vi "CSS grouping with jaccard index.vi"() -> ()   [LabVIEW 2014]
uses:
  <vilib>/Utility/file.llb/Read From Spreadsheet File (string).vi
  <vilib>/Utility/file.llb/Write To Spreadsheet File (string).vi
panel:
  in  "save":bool
  in  "file path (to write) 2":path
  in  "cycles":i32=1
  out "Array":string[](array[string])
  in  "cluster centers (original) 7":string[](array[string])=["0 -1 1 -4 0", "0 -1 2 -2 0", "0 -2 3 -3 0", "0 -3 4 -4 0", "0 -1 1 -4 4 -3 0", "0 -1 2 -2 3 -3 0", "0 -4 1 -1 2 -2 0", "0 -4 4 -3 3 -2 0", "0 -1 1 -4 0 -2 3 -3 0", "0 -1 2 -2 0 -4 4 -3 0"]
  out "Assignment (enhanced)":string[](array[string])
  out "Assignment":string[](array[string])
  out "all rows":string[][](array[string])
  in  "cluster centers (original) 5":string[](array[string])=["0 -1 1 -4 0 -4 1 -1 0 -1 1 -4 0 -4 1 -1 0 -1 1 -4 0 -4 1 -1 0 -1 0 -1 1 -4 0 -4 1 -1 0", "0 -1 2 -2 0 -2 2 -1 0 -1 2 -2 0 -2 2 -1 0 -1 2 -2 0 -2 2 -1 0 -1 0 -1 2 -2 0 -2 2 -1 0", "0 -2 3 -3 0 -3 3 -2 0 -2 3 -3 0 -3 3 -2 0 -2 3 -3 0 -3 3 -2 0 -2 0 -2 3 -3 0 -3 3 -2 0", "0 -3 4 -4 0 -4 4 -3 0 -3 4 -4 0 -4 4 -3 0 -3 4 -4 0 -4 4 -3 0 -3 0 -3 4 -4 0 -4 4 -3 0", "0 -1 1 -4 4 -3 0 -3 4 -4 1 -1 0 -1 1 -4 4 -3 0 -3 4 -4 1 -1 0 -1 1 -4 4 -3 0 -3 4 -4 1 -1 0 -1 1 -4 4 -3 0 -3 4 -4 1 -1 0", "0 -1 2 -2 3 -3 0 -3 3 -2 2 -1 0 -1 2 -2 3 -3 0 -3 3 -2 2 -1 0 -1 2 -2 3 -3 0 -3 3 -2 2 -1 0 -1 2 -2 3 -3 0 -3 3 -2 2 -1 0", "0 -4 1 -1 2 -2 0 -2 2 -1 1 -4 0 -4 1 -1 2 -2 0 -2 2 -1 1 -4 0 -4 1 -1 2 -2 0 -2 2 -1 1 -4 0 -4 1 -1 2 -2 0 -2 2 -1 1 -4 0", "0 -4 4 -3 3 -2 0 -2 3 -3 4 -4 0 -4 4 -3 3 -2 0 -2 3 -3 4 -4 0 -4 4 -3 3 -2 0 -2 3 -3 4 -4 0 -4 4 -3 3 -2 0 -2 3 -3 4 -4 0", "0 -1 1 -4 0 -2 3 -3 0 -3 3 -2 0 -4 1 -1 0 -1 1 -4 0 -2 3 -3 0 -3 3 -2 0 -4 1 -1 0 -1 1 -4 0 -2 3 -3 0 -3 3 -2 0 -4 1 -1 0 -1 1 -4 0 -2 3 -3 0 -3 3 -2 0 -4 1 -1 0", "0 -1 2 -2 0 -4 4 -3 0 -3 4 -4 0 -2 2 -1 0 -1 2 -2 0 -4 4 -3 0 -3 4 -4 0 -2 2 -1 0 -1 2 -2 0 -4 4 -3 0 -3 4 -4 0 -2 2 -1 0 -1 2 -2 0 -4 4 -3 0 -3 4 -4 0 -2 2 -1 0"]
  in  "cluster centers (original) 4":string[](array[string])=["0 -1 1 -4 0 -4 1 -1 0 -1 1 -4 0 -4 1 -1 0", "0 -1 2 -2 0 -2 2 -1 0 -1 2 -2 0 -2 2 -1 0", "0 -2 3 -3 0 -3 3 -2 0 -2 3 -3 0 -3 3 -2 0", "0 -3 4 -4 0 -4 4 -3 0 -3 4 -4 0 -4 4 -3 0", "0 -1 1 -4 4 -3 0 -3 4 -4 1 -1 0 -1 1 -4 4 -3 0 -3 4 -4 1 -1 0", "0 -1 2 -2 3 -3 0 -3 3 -2 2 -1 0 -1 2 -2 3 -3 0 -3 3 -2 2 -1 0", "0 -4 1 -1 2 -2 0 -2 2 -1 1 -4 0 -4 1 -1 2 -2 0 -2 2 -1 1 -4 0", "0 -4 4 -3 3 -2 0 -2 3 -3 4 -4 0 -4 4 -3 3 -2 0 -2 3 -3 4 -4 0", "0 -1 1 -4 0 -2 3 -3 0 -3 3 -2 0 -4 1 -1 0 -1 1 -4 0 -2 3 -3 0 -3 3 -2 0 -4 1 -1 0", "0 -1 2 -2 0 -4 4 -3 0 -3 4 -4 0 -2 2 -1 0 -1 2 -2 0 -4 4 -3 0 -3 4 -4 0 -2 2 -1 0"]
  out "size(s)":i32
  in  "cluster centers (original) 3":string[](array[string])=["0 -1 1 -4 0 -4 1 -1 0 -1 1 -4 0 -4 1 -1 0 -1 1 -4 0 -4 1 -1 0", "0 -1 2 -2 0 -2 2 -1 0 -1 2 -2 0 -2 2 -1 0 -1 2 -2 0 -2 2 -1 0", "0 -2 3 -3 0 -3 3 -2 0 -2 3 -3 0 -3 3 -2 0 -2 3 -3 0 -3 3 -2 0", "0 -3 4 -4 0 -4 4 -3 0 -3 4 -4 0 -4 4 -3 0 -3 4 -4 0 -4 4 -3 0", "0 -1 1 -4 4 -3 0 -3 4 -4 1 -1 0 -1 1 -4 4 -3 0 -3 4 -4 1 -1 0 -1 1 -4 4 -3 0 -3 4 -4 1 -1 0", "0 -1 2 -2 3 -3 0 -3 3 -2 2 -1 0 -1 2 -2 3 -3 0 -3 3 -2 2 -1 0 -1 2 -2 3 -3 0 -3 3 -2 2 -1 0", "0 -4 1 -1 2 -2 0 -2 2 -1 1 -4 0 -4 1 -1 2 -2 0 -2 2 -1 1 -4 0 -4 1 -1 2 -2 0 -2 2 -1 1 -4 0", "0 -4 4 -3 3 -2 0 -2 3 -3 4 -4 0 -4 4 -3 3 -2 0 -2 3 -3 4 -4 0 -4 4 -3 3 -2 0 -2 3 -3 4 -4 0", "0 -1 1 -4 0 -2 3 -3 0 -3 3 -2 0 -4 1 -1 0 -1 1 -4 0 -2 3 -3 0 -3 3 -2 0 -4 1 -1 0 -1 1 -4 0 -2 3 -3 0 -3 3 -2 0 -4 1 -1 0", "0 -1 2 -2 0 -4 4 -3 0 -3 4 -4 0 -2 2 -1 0 -1 2 -2 0 -4 4 -3 0 -3 4 -4 0 -2 2 -1 0 -1 2 -2 0 -4 4 -3 0 -3 4 -4 0 -2 2 -1 0"]
  in  "cluster centers (original) 2":string[](array[string])=["0 -1 1 -4 0 -4 1 -1 0", "0 -1 2 -2 0 -2 2 -1 0", "0 -2 3 -3 0 -3 3 -2 0", "0 -3 4 -4 0 -4 4 -3 0", "0 -1 1 -4 4 -3 0 -3 4 -4 1 -1 0", "0 -1 2 -2 3 -3 0 -3 3 -2 2 -1 0", "0 -4 1 -1 2 -2 0 -2 2 -1 1 -4 0", "0 -4 4 -3 3 -2 0 -2 3 -3 4 -4 0", "0 -1 1 -4 0 -2 3 -3 0 -3 3 -2 0 -4 1 -1 0", "0 -1 2 -2 0 -4 4 -3 0 -3 4 -4 0 -2 2 -1 0"]
  out "accuracy":string[][](array[string])
  in  "cluster centers (original) long 5":string[](array[string])=["1 0 -1 1 -1 0 -4 1 -4 0 1 0 -1 1 -1 0 -4 1 -4 0 1 0 -1 1 -1 0 -4 1 -4 0 1 0 -1 1 -1 0 -4 1 -4 0 1 0 -1 1 -1 0 -4 1 -4 0 1", "2 0 -1 2 -1 0 -2 2 -2 0 2 0 -1 2 -1 0 -2 2 -2 0 2 0 -1 2 -1 0 -2 2 -2 0 2 0 -1 2 -1 0 -2 2 -2 0 2 0 -1 2 -1 0 -2 2 -2 0 2", "3 0 -3 3 -3 0 -2 3 -2 0 3 0 -3 3 -3 0 -2 3 -2 0 3 0 -3 3 -3 0 -2 3 -2 0 3 0 -3 3 -3 0 -2 3 -2 0 3 0 -3 3 -3 0 -2 3 -2 0 3", "4 0 -3 4 -3 0 -4 4 -4 0 4 0 -3 4 -3 0 -4 4 -4 0 4 0 -3 4 -3 0 -4 4 -4 0 4 0 -3 4 -3 0 -4 4 -4 0 4 0 -3 4 -3 0 -4 4 -4 0 4", "-1 1 -4 0 -4 4 -3 4 -4 0 -4 1 -1 1 -4 0 -4 4 -3 4 -4 0 -4 1 -1 1 -4 0 -4 4 -3 4 -4 0 -4 1 -1 1 -4 0 -4 4 -3 4 -4 0 -4 1 -1 1 -4 0 -4 4 -3 4 -4 0 -4 1 -1", "-1 2 -2 0 -2 3 -3 3 -2 0 -2 2 -1 2 -2 0 -2 3 -3 3 -2 0 -2 2 -1 2 -2 0 -2 3 -3 3 -2 0 -2 2 -1 2 -2 0 -2 3 -3 3 -2 0 -2 2 -1 2 -2 0 -2 3 -3 3 -2 0 -2 2 -1", "-4 1 -1 0 -1 2 -2 2 -1 0 -1 1 -4 1 -1 0 -1 2 -2 2 -1 0 -1 1 -4 1 -1 0 -1 2 -2 2 -1 0 -1 1 -4 1 -1 0 -1 2 -2 2 -1 0 -1 1 -4 1 -1 0 -1 2 -2 2 -1 0 -1 1 -4", "-4 4 -3 0 -3 3 -2 3 -3 0 -3 4 -4 4 -3 0 -3 3 -2 3 -3 0 -3 4 -4 4 -3 0 -3 3 -2 3 -3 0 -3 4 -4 4 -3 0 -3 3 -2 3 -3 0 -3 4 -4 4 -3 0 -3 3 -2 3 -3 0 -3 4 -4", "0 -4 1 -1 0 -3 3 -2 3 -3 0 -1 1 -4 0 -4 1 -1 0 -3 3 -2 3 -3 0 -1 1 -4 0 -4 1 -1 0 -3 3 -2 3 -3 0 -1 1 -4 0 -4 1 -1 0 -3 3 -2 3 -3 0 -1 1 -4 0 -4 1 -1 0 -3 3 -2 3 -3 0 -1 1 -4 0", "0 -4 4 -3 0 -1 2 -2 2 -1 0 -3 4 -4 0 -4 4 -3 0 -1 2 -2 2 -1 0 -3 4 -4 0 -4 4 -3 0 -1 2 -2 2 -1 0 -3 4 -4 0 -4 4 -3 0 -1 2 -2 2 -1 0 -3 4 -4 0 -4 4 -3 0 -1 2 -2 2 -1 0 -3 4 -4 0"]
  in  "cluster centers (original) long 4":string[](array[string])=["1 0 -1 1 -1 0 -4 1 -4 0 1 0 -1 1 -1 0 -4 1 -4 0 1 0 -1 1 -1 0 -4 1 -4 0 1 0 -1 1 -1 0 -4 1 -4 0 1", "2 0 -1 2 -1 0 -2 2 -2 0 2 0 -1 2 -1 0 -2 2 -2 0 2 0 -1 2 -1 0 -2 2 -2 0 2 0 -1 2 -1 0 -2 2 -2 0 2", "3 0 -3 3 -3 0 -2 3 -2 0 3 0 -3 3 -3 0 -2 3 -2 0 3 0 -3 3 -3 0 -2 3 -2 0 3 0 -3 3 -3 0 -2 3 -2 0 3", "4 0 -3 4 -3 0 -4 4 -4 0 4 0 -3 4 -3 0 -4 4 -4 0 4 0 -3 4 -3 0 -4 4 -4 0 4 0 -3 4 -3 0 -4 4 -4 0 4", "-1 1 -4 0 -4 4 -3 4 -4 0 -4 1 -1 1 -4 0 -4 4 -3 4 -4 0 -4 1 -1 1 -4 0 -4 4 -3 4 -4 0 -4 1 -1 1 -4 0 -4 4 -3 4 -4 0 -4 1 -1", "-1 2 -2 0 -2 3 -3 3 -2 0 -2 2 -1 2 -2 0 -2 3 -3 3 -2 0 -2 2 -1 2 -2 0 -2 3 -3 3 -2 0 -2 2 -1 2 -2 0 -2 3 -3 3 -2 0 -2 2 -1", "-4 1 -1 0 -1 2 -2 2 -1 0 -1 1 -4 1 -1 0 -1 2 -2 2 -1 0 -1 1 -4 1 -1 0 -1 2 -2 2 -1 0 -1 1 -4 1 -1 0 -1 2 -2 2 -1 0 -1 1 -4", "-4 4 -3 0 -3 3 -2 3 -3 0 -3 4 -4 4 -3 0 -3 3 -2 3 -3 0 -3 4 -4 4 -3 0 -3 3 -2 3 -3 0 -3 4 -4 4 -3 0 -3 3 -2 3 -3 0 -3 4 -4", "0 -4 1 -1 0 -3 3 -2 3 -3 0 -1 1 -4 0 -4 1 -1 0 -3 3 -2 3 -3 0 -1 1 -4 0 -4 1 -1 0 -3 3 -2 3 -3 0 -1 1 -4 0 -4 1 -1 0 -3 3 -2 3 -3 0 -1 1 -4 0", "0 -4 4 -3 0 -1 2 -2 2 -1 0 -3 4 -4 0 -4 4 -3 0 -1 2 -2 2 -1 0 -3 4 -4 0 -4 4 -3 0 -1 2 -2 2 -1 0 -3 4 -4 0 -4 4 -3 0 -1 2 -2 2 -1 0 -3 4 -4 0"]
  in  "cluster centers (original) long 3":string[](array[string])=["1 0 -1 1 -1 0 -4 1 -4 0 1 0 -1 1 -1 0 -4 1 -4 0 1 0 -1 1 -1 0 -4 1 -4 0 1", "2 0 -1 2 -1 0 -2 2 -2 0 2 0 -1 2 -1 0 -2 2 -2 0 2 0 -1 2 -1 0 -2 2 -2 0 2", "3 0 -3 3 -3 0 -2 3 -2 0 3 0 -3 3 -3 0 -2 3 -2 0 3 0 -3 3 -3 0 -2 3 -2 0 3", "4 0 -3 4 -3 0 -4 4 -4 0 4 0 -3 4 -3 0 -4 4 -4 0 4 0 -3 4 -3 0 -4 4 -4 0 4", "-1 1 -4 0 -4 4 -3 4 -4 0 -4 1 -1 1 -4 0 -4 4 -3 4 -4 0 -4 1 -1 1 -4 0 -4 4 -3 4 -4 0 -4 1 -1", "-1 2 -2 0 -2 3 -3 3 -2 0 -2 2 -1 2 -2 0 -2 3 -3 3 -2 0 -2 2 -1 2 -2 0 -2 3 -3 3 -2 0 -2 2 -1", "-4 1 -1 0 -1 2 -2 2 -1 0 -1 1 -4 1 -1 0 -1 2 -2 2 -1 0 -1 1 -4 1 -1 0 -1 2 -2 2 -1 0 -1 1 -4", "-4 4 -3 0 -3 3 -2 3 -3 0 -3 4 -4 4 -3 0 -3 3 -2 3 -3 0 -3 4 -4 4 -3 0 -3 3 -2 3 -3 0 -3 4 -4", "0 -4 1 -1 0 -3 3 -2 3 -3 0 -1 1 -4 0 -4 1 -1 0 -3 3 -2 3 -3 0 -1 1 -4 0 -4 1 -1 0 -3 3 -2 3 -3 0 -1 1 -4 0", "0 -4 4 -3 0 -1 2 -2 2 -1 0 -3 4 -4 0 -4 4 -3 0 -1 2 -2 2 -1 0 -3 4 -4 0 -4 4 -3 0 -1 2 -2 2 -1 0 -3 4 -4 0"]
  in  "cluster centers (original) long":string[](array[string])=["1 0 -1 1 -1 0 -4 1 -4 0 1 0 -1 1 -1 0 -4 1 -4 0 1", "2 0 -1 2 -1 0 -2 2 -2 0 2 0 -1 2 -1 0 -2 2 -2 0 2", "3 0 -3 3 -3 0 -2 3 -2 0 3 0 -3 3 -3 0 -2 3 -2 0 3", "4 0 -3 4 -3 0 -4 4 -4 0 4 0 -3 4 -3 0 -4 4 -4 0 4", "-1 1 -4 0 -4 4 -3 4 -4 0 -4 1 -1 1 -4 0 -4 4 -3 4 -4 0 -4 1 -1", "-1 2 -2 0 -2 3 -3 3 -2 0 -2 2 -1 2 -2 0 -2 3 -3 3 -2 0 -2 2 -1", "-4 1 -1 0 -1 2 -2 2 -1 0 -1 1 -4 1 -1 0 -1 2 -2 2 -1 0 -1 1 -4", "-4 4 -3 0 -3 3 -2 3 -3 0 -3 4 -4 4 -3 0 -3 3 -2 3 -3 0 -3 4 -4", "0 -4 1 -1 0 -3 3 -2 3 -3 0 -1 1 -4 0 -4 1 -1 0 -3 3 -2 3 -3 0 -1 1 -4 0", "0 -4 4 -3 0 -1 2 -2 2 -1 0 -3 4 -4 0 -4 4 -3 0 -1 2 -2 2 -1 0 -3 4 -4 0"]
  out "Results":string[][](array[string])
  in  "file path (dialog if empty)":path=path "K:/PhD work/PhD research work 2/Common substring validation/documentation/Data final results/Common substrings (ground truth 2 CHECKED).txt"
  in  "cluster centers (original)":string[](array[string])=["1 0 -1 1 -1 0 -4 1 -4 0 1", "2 0 -1 2 -1 0 -2 2 -2 0 2", "3 0 -3 3 -3 0 -2 3 -2 0 3", "4 0 -3 4 -3 0 -4 4 -4 0 4", "-1 1 -4 0 -4 4 -3 4 -4 0 -4 1 -1", "-1 2 -2 0 -2 3 -3 3 -2 0 -2 2 -1", "-4 1 -1 0 -1 2 -2 2 -1 0 -1 1 -4", "-4 4 -3 0 -3 3 -2 3 -3 0 -3 4 -4", "0 -4 1 -1 0 -3 3 -2 3 -3 0 -1 1 -4 0", "0 -4 4 -3 0 -1 2 -2 2 -1 0 -3 4 -4 0"]
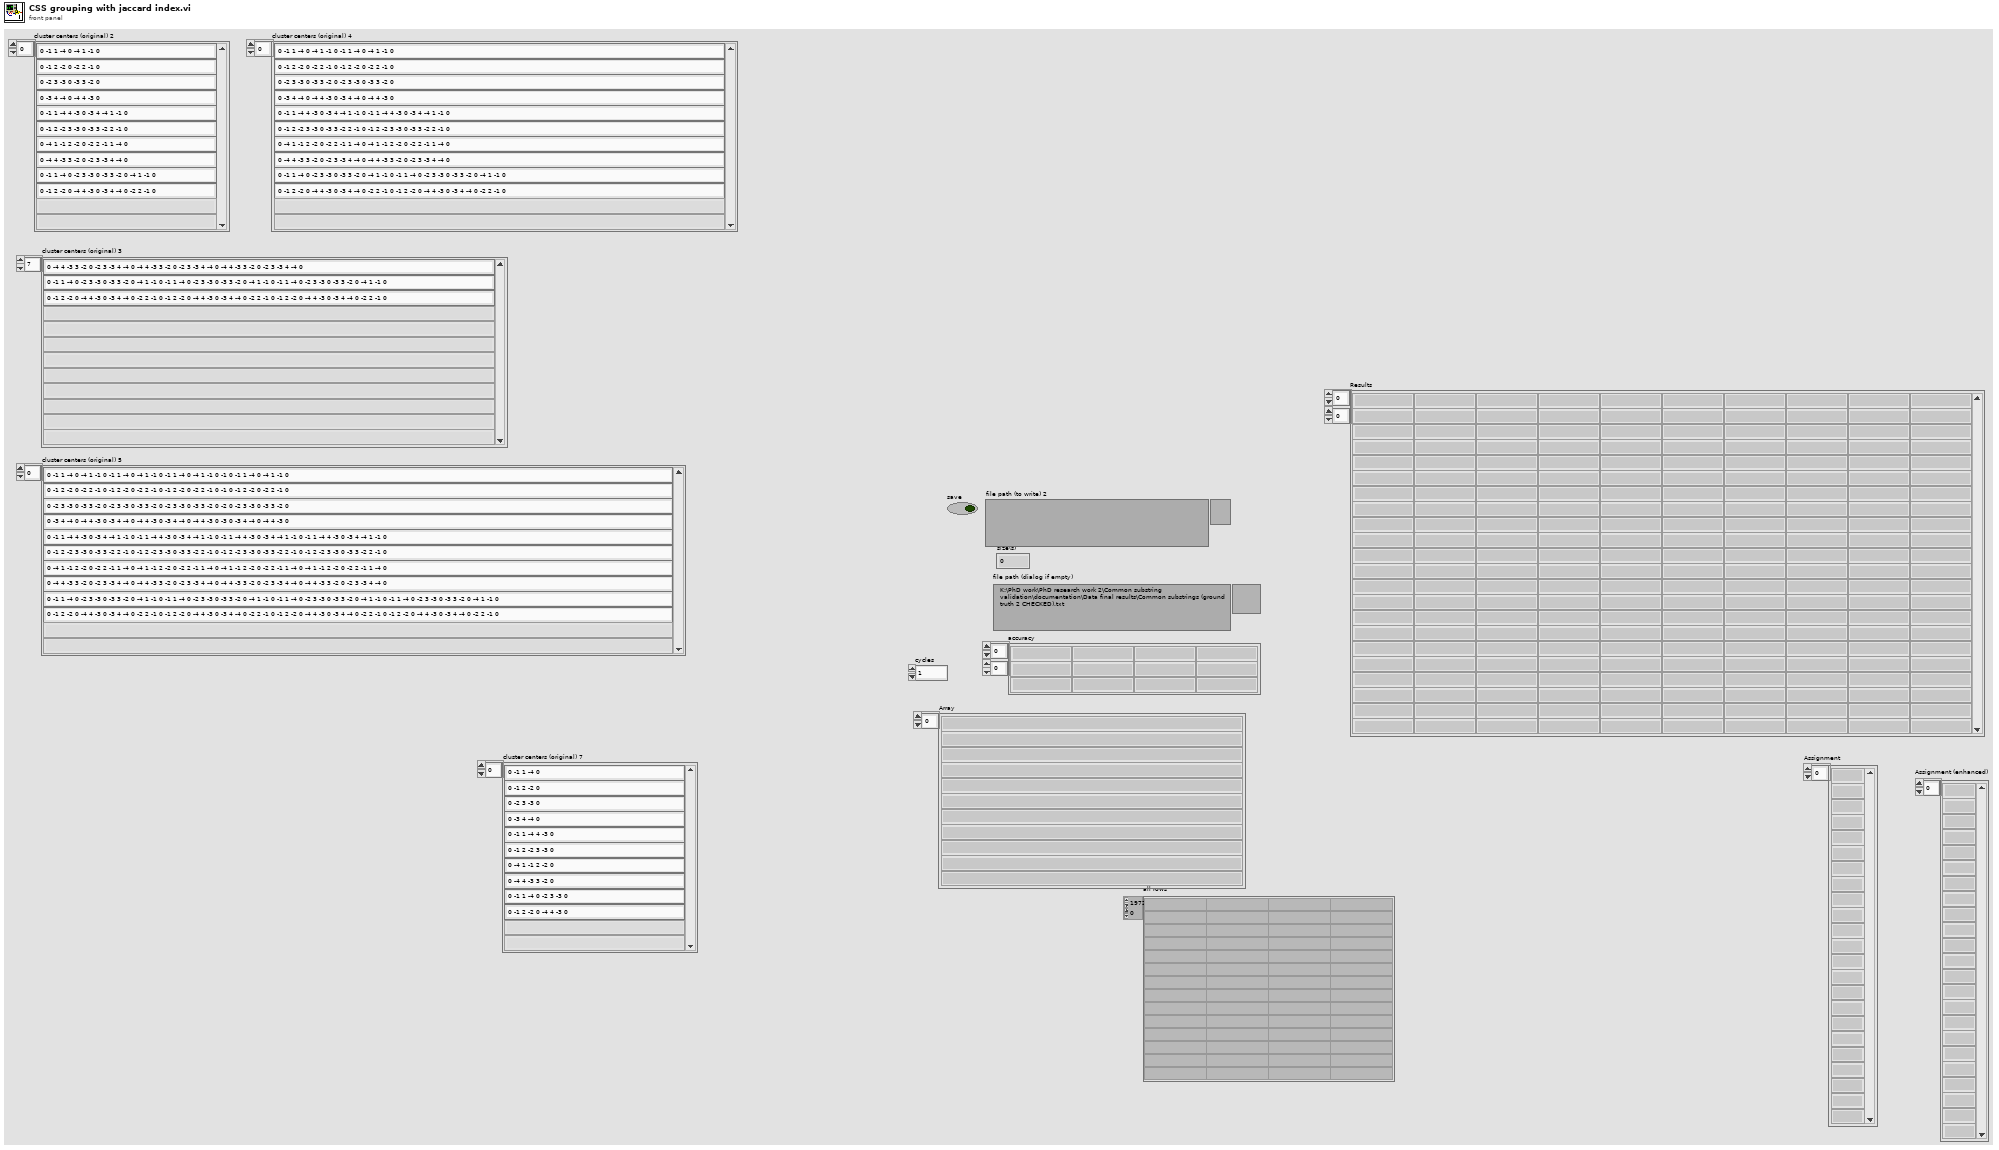
[diagram p1: front panel]
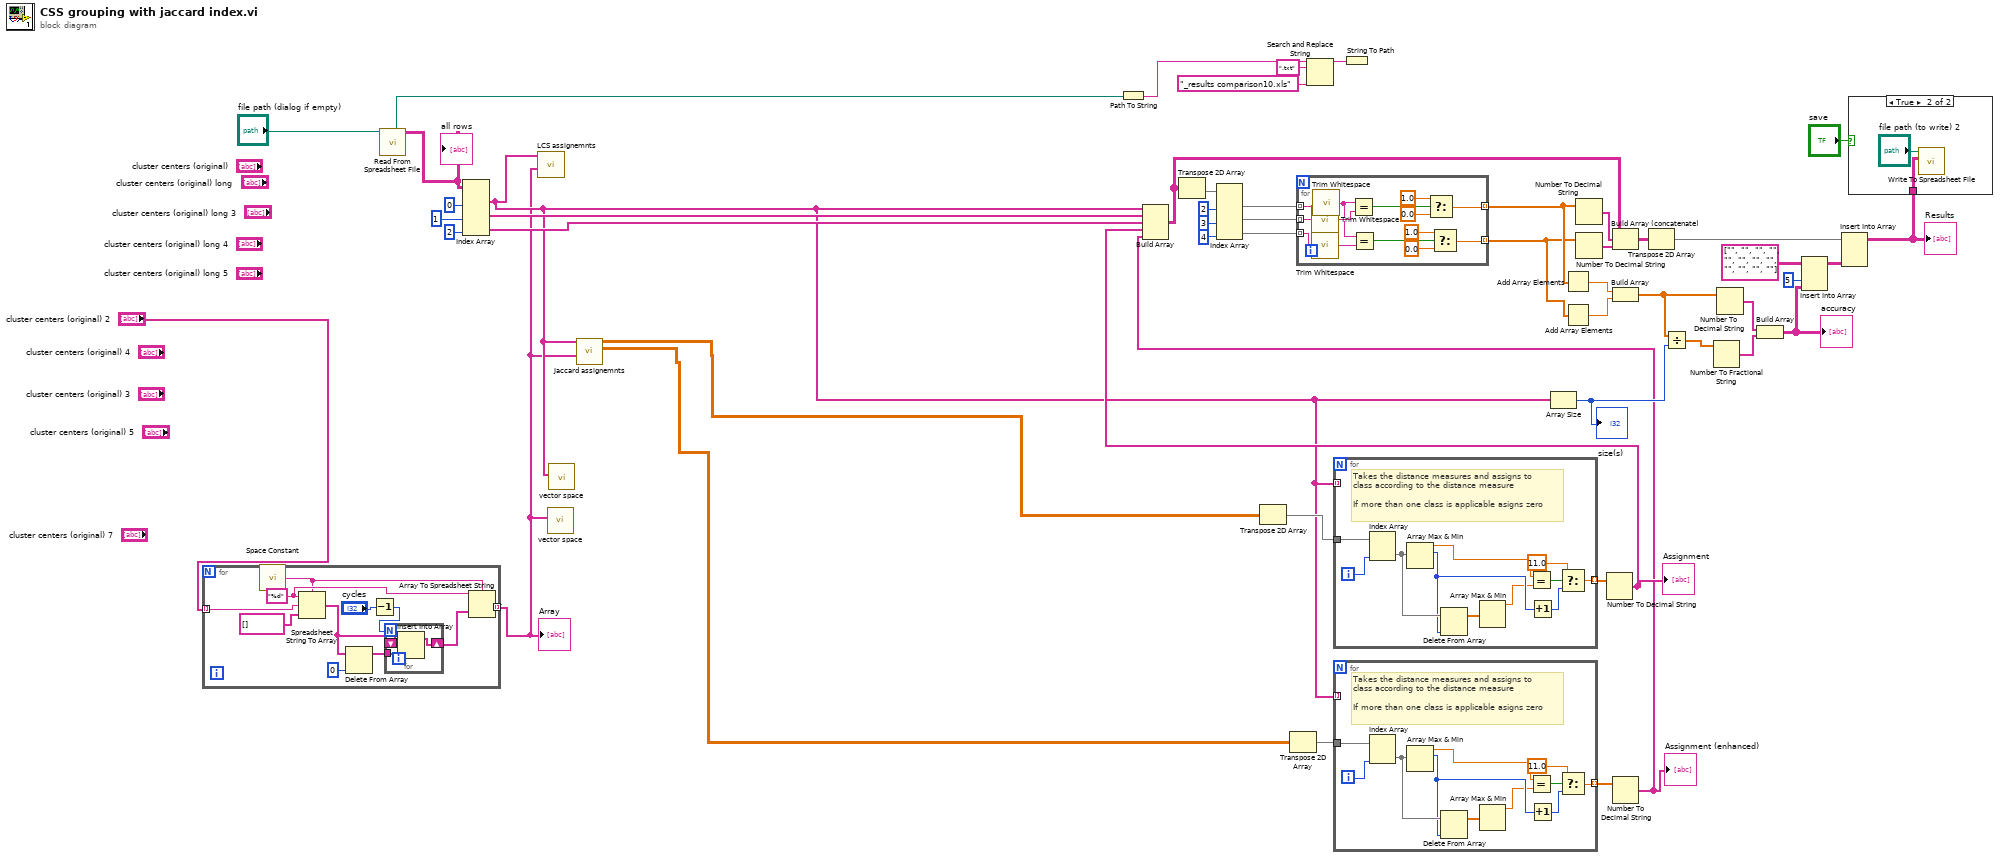
[diagram p0: block diagram]
diagram:
  n1 = for {
    tunnel: "cluster centers (original) 2" -> [w60] mode=indexing
    tunnel: [w54] -> w7 mode=indexing
    w55 = "%d" ("format string")
    n2 = call <vilib>:"Space Constant.vi"() -> ("String"=w53:string)
    n3 = Spreadsheet String To Array(delimiter (Tab)=w53, format string=w55, spreadsheet string=w60, array type (2D Dbl)=string[] []) -> (array=w58:string[])
    n4 = Delete From Array(array=w58, index=0) -> (array with subset deleted=w57:string[])  [unwired: 1 in, 1 out]
    n5 = Decrement(x="cycles") -> (x-1=w52:i32)
    n6 = for {
      N: w52 -> [_]
      tunnel: w57 -> [w63]
      shift-right: [w62] -> w56
      shift-left: w58 -> [w64]
      n7 = Insert Into Array(array=w64, new element=w63) -> (w62:string[])  [unwired: 1 in]
    }
    n8 = Array To Spreadsheet String(delimiter (Tab)=w53, array=w56, 3:w55) -> (spreadsheet string=w54:string)
  }
  "Array" <- w7
  n9 = call-poly <vilib>:"Read From Spreadsheet File.vi"("file path (dialog if empty)"="file path (dialog if empty)") -> ("all rows"=w2:string[][], "new file path (Not A Path if cancelled)"=w48:path)  [unwired: 6 in, 3 out]
  "all rows" <- w2
  n10 = Index Array(array=w2, index (col) #1=0 ("disabled index (col)"), index (col) #2=1 ("index (col)"), index (col) #3=2 ("index (col)")) -> (element #1=w8:string[], element #2=w16:string[], element #3=w15:string[])  [unwired: 3 in]
  n11 = call "LCS assignemnts.vi"("cluster centers"=w7, "Patterns in"=w8) -> ()  [unwired: 1 in, 9 out]
  n12 = call "vector space.vi"("Full transition sequence from service to end"=w7) -> ()  [unwired: 8 in, 3 out]
  n13 = call "vector space.vi"("Full transition sequence from service to end"=w8) -> ()  [unwired: 8 in, 3 out]
  n14 = call "Jaccard assignemnts.vi"("cluster centers in"=w7, "patterns in"=w8) -> ("distance values out enhanced (set)"=w3:dbl[][], "distance values out (set)"=w4:dbl[][])  [unwired: 6 in, 2 out]
  n15 = Path To String(path=w48) -> (string=w47:string)
  n16 = Transpose 2D Array(2D array=w4) -> (transposed array=w13:dbl[][])
  n17 = Transpose 2D Array(2D array=w3) -> (transposed array=w10:dbl[][])
  n18 = Search and Replace String(input string=w47, search string=".txt", replace string="_results comparison10.xls" ("replace string (\"\")")) -> (result string=w44:string)  [unwired: 5 in, 3 out]
  n19 = for {
    tunnel: w13 -> [w75]
    tunnel: [w65] -> w14 mode=indexing
    tunnel: w8 -> [_] mode=indexing
    i -> [w74]
    # "Takes the distance measures and assigns to \nclass according to the distance measure\n\nIf more than one class is applicable asigns zero"
    n20 = Index Array(array=w75, index (col)=w74) -> (element=w69:dbl[])  [unwired: 1 in]
    n21 = Array Max & Min(array=w69) -> (max value=w68:dbl, max index (indices)=w67:i32)  [unwired: 2 out]
    n22 = Delete From Array(array=w69, index=w67) -> (array with subset deleted=w73:dbl[])  [unwired: 1 in, 1 out]
    n23 = Array Max & Min(array=w73) -> (max value=w66:dbl)  [unwired: 3 out]
    n24 = Equal?(x=w68, y=w66) -> (x = y?=w72:bool)
    n25 = Increment(x=w67) -> (x+1=w70:i32)
    n26 = Select(t=11.0, s=w72, f=w70) -> (s? t:f=w65:dbl)
  }
  n27 = for {
    tunnel: w10 -> [w86]
    tunnel: [w76] -> w11 mode=indexing
    tunnel: w8 -> [_] mode=indexing
    i -> [w85]
    # "Takes the distance measures and assigns to \nclass according to the distance measure\n\nIf more than one class is applicable asigns zero"
    n28 = Index Array(array=w86, index (col)=w85) -> (element=w80:dbl[])  [unwired: 1 in]
    n29 = Array Max & Min(array=w80) -> (max value=w79:dbl, max index (indices)=w78:i32)  [unwired: 2 out]
    n30 = Delete From Array(array=w80, index=w78) -> (array with subset deleted=w84:dbl[])  [unwired: 1 in, 1 out]
    n31 = Array Max & Min(array=w84) -> (max value=w77:dbl)  [unwired: 3 out]
    n32 = Equal?(x=w79, y=w77) -> (x = y?=w83:bool)
    n33 = Increment(x=w78) -> (x+1=w81:i32)
    n34 = Select(t=11.0, s=w83, f=w81) -> (s? t:f=w76:dbl)
  }
  n35 = String To Path(string=w44) -> ()  [unwired: 1 out]
  n36 = Array Size(array=w8) -> (size(s)=w17:i32)
  "size(s)" <- w17
  n37 = Number To Decimal String(number=w14) -> (decimal integer string=w12:string[])  [unwired: 1 in]
  "Assignment" <- w12
  n38 = Number To Decimal String(number=w11) -> (decimal integer string=w9:string[])  [unwired: 1 in]
  "Assignment (enhanced)" <- w9
  n39 = Build Array(w8, w16, w15, w12, w9) -> (w33:string[][])
  n40 = Transpose 2D Array(2D array=w33) -> (transposed array=w36:string[][])
  n41 = Index Array(array=w36, index (col) #1=2 ("disabled index (col)"), index (col) #2=3 ("index (col)"), index (col) #3=4 ("index (col)")) -> (element #1=w39:string[], element #2=w38:string[], element #3=w37:string[])  [unwired: 3 in]
  n42 = for {
    tunnel: w39 -> [w92] mode=indexing
    tunnel: w38 -> [w91] mode=indexing
    tunnel: w37 -> [w90] mode=indexing
    tunnel: [w94] -> w20 mode=indexing
    tunnel: [w93] -> w19 mode=indexing
    n43 = call <vilib>:"Trim Whitespace.vi"("string"=w91) -> ("trimmed string"=w89:string)  [unwired: 1 in]
    n44 = call <vilib>:"Trim Whitespace.vi"("string"=w90) -> ("trimmed string"=w88:string)  [unwired: 1 in]
    n45 = call <vilib>:"Trim Whitespace.vi"("string"=w92) -> ("trimmed string"=w87:string)  [unwired: 1 in]
    n46 = Equal?(x=w87, y=w89) -> (x = y?=w100:bool)
    n47 = Equal?(x=w87, y=w88) -> (x = y?=w95:bool)
    n48 = Select(t=1.0, s=w100, f=0.0) -> (s? t:f=w94:dbl)
    n49 = Select(t=1.0, s=w95, f=0.0) -> (s? t:f=w93:dbl)
  }
  n50 = Add Array Elements(numeric array=w20) -> (sum=w21:dbl)
  n51 = Add Array Elements(numeric array=w19) -> (sum=w22:dbl)
  n52 = Number To Decimal String(number=w20) -> (decimal integer string=w35:string[])  [unwired: 1 in]
  n53 = Number To Decimal String(number=w19) -> (decimal integer string=w34:string[])  [unwired: 1 in]
  n54 = Build Array (concatenate)(w33, w35, w34) -> (w32:string[][])
  n55 = Build Array(w21, w22) -> (w23:dbl[])
  n56 = Transpose 2D Array(2D array=w32) -> (transposed array=w18:string[][])
  n57 = Divide(x=w23, y=w17) -> (x/y=w24:dbl[])
  n58 = Number To Fractional String(number=w24) -> (F-format string=w26:string[])  [unwired: 3 in]
  n59 = Number To Decimal String(number=w23) -> (decimal integer string=w25:string[])  [unwired: 1 in]
  n60 = Build Array(w25, w26) -> (w30:string[][])
  "accuracy" <- w30
  n61 = Insert Into Array(array=string[][] [["", "", "", "", "", ""], ["", "", "", "", "", ""]] ("appended array 3"), index (col)=5 ("disabled index (col)"), new element=w30) -> (w29:string[][])  [unwired: 1 in]
  n62 = Insert Into Array(array=w18, new element=w29) -> (w6:string[][])  [unwired: 2 in]
  "Results" <- w6
  n63 = case shown="True" "save" {
    tunnel: w6 -> [_ w101]
    frame False {
    }
    frame True {
      n64 = call-poly <vilib>:"Write To Spreadsheet File.vi"("2D data"=w101, "file path (dialog if empty)"="file path (to write) 2") -> ()  [unwired: 6 in, 1 out]
    }
  }
